vi "CalcPress.vi"(8 "error in (no error)":errorcluster, 10 "Adc_press":i32, 11 "BME68x in":refnum<class "BME680.lvclass">) -> (0 "error out":errorcluster, 2 "Press":i32, 3 "BME68x out":refnum<class "BME680.lvclass">)   [LabVIEW 2022 SP3, in "BME680.lvlib" / "BME680.lvclass"]
uses:
  BME680.lvclass
  BME680.lvclass/BME680.ctl
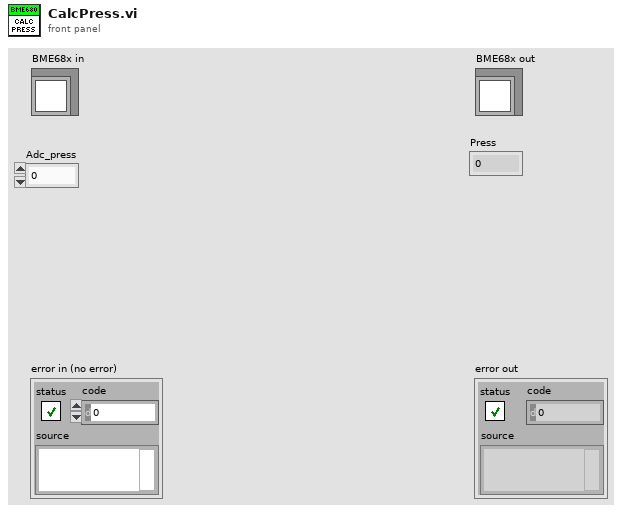
[diagram p1: front panel]
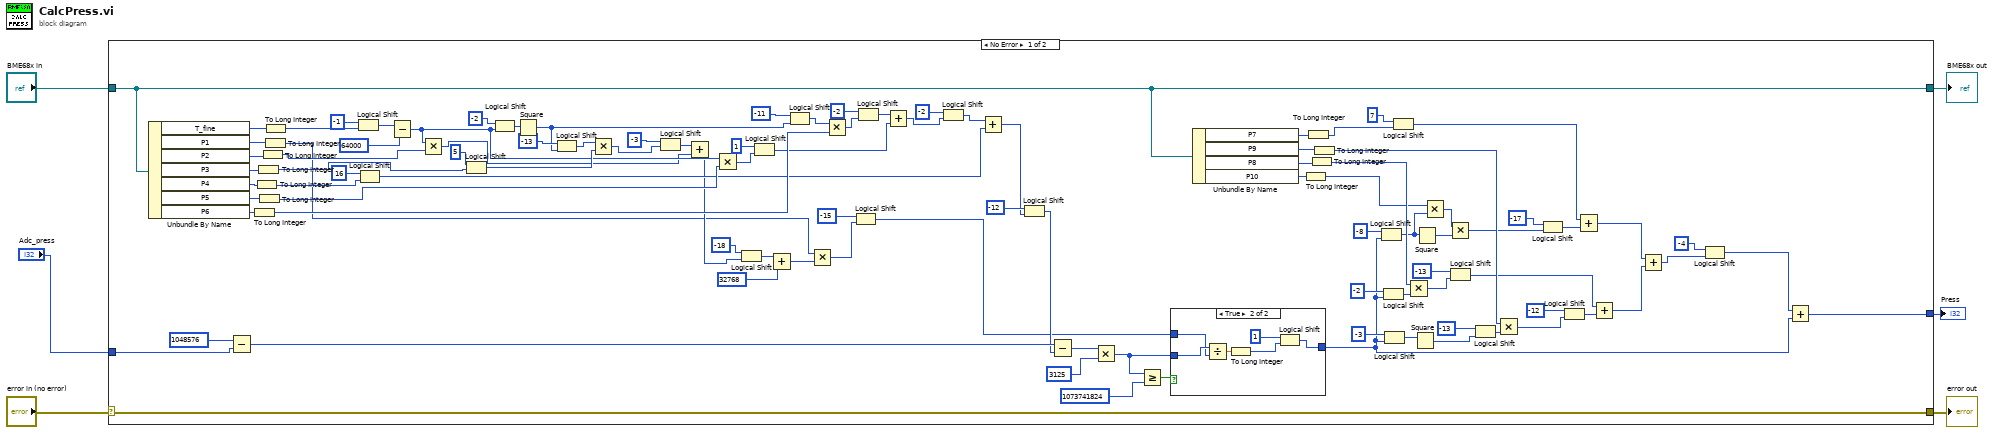
[diagram p0: block diagram]
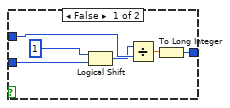
[diagram p2: hidden frame]
diagram:
  n1 = case shown="No Error" "error in (no error)" {
    selector: "error in (no error)" -> [w106 w120]
    tunnel: [w106 w120] -> w5
    tunnel: [w8 w119] -> w3
    tunnel: "BME68x in" -> [w8 w119]
    tunnel: "Adc_press" -> [w55 _]
    tunnel: [w7 _] -> w1
    frame No Error {
      n2 = Unbundle By Name(w8) -> ("T_fine"=w104:i32, "P1"=w105:u16, "P2"=w77:u16, "P3"=w78:u8, "P4"=w82:u16, "P5"=w92:u16, "P6"=w96:u8)
      n3 = Subtract(x=1048576 ("y"), y=w55) -> (x-y=w54:i32)
      n4 = To Long Integer(number=w96) -> (32bit integer=w93:i32)
      n5 = To Long Integer(number=w82) -> (32bit integer=w80:i32)
      n6 = To Long Integer(number=w78) -> (32bit integer=w73:i32)
      n7 = To Long Integer(number=w92) -> (32bit integer=w88:i32)
      n8 = To Long Integer(number=w77) -> (32bit integer=w68:i32)
      n9 = To Long Integer(number=w105) -> (32bit integer=w60:i32)
      n10 = To Long Integer(number=w104) -> (32bit integer=w103:i32)
      n11 = Logical Shift(y=i16 -1, x=w103) -> (x << y=w101:i32)
      n12 = Logical Shift(y=i16 16, x=w80) -> (x << y=w79:i32)
      n13 = Subtract(x=w101, y=64000) -> (x-y=w67:i32)
      n14 = Multiply(x=w67, y=w68) -> (x*y=w65:i32)
      n15 = Logical Shift(y=i16 5, x=w73) -> (x << y=w72:i32)
      n16 = Logical Shift(y=i16 -2, x=w67) -> (x << y=w98:i32)
      n17 = Square(x=w98) -> (x^2=w75:i32)
      n18 = Logical Shift(y=i16 -13, x=w75) -> (x << y=w71:i32)
      n19 = Multiply(x=w71, y=w72) -> (x*y=w69:i32)
      n20 = Logical Shift(y=i16 -3, x=w69) -> (x << y=w66:i32)
      n21 = Add(x=w66, y=w65) -> (x+y=w63:i32)
      n22 = Multiply(x=w67, y=w88) -> (x*y=w87:i32)
      n23 = Logical Shift(y=i16 -18, x=w63) -> (x << y=w62:i32)
      n24 = Logical Shift(y=i16 1, x=w87) -> (x << y=w86:i32)
      n25 = Add(x=w62, y=32768) -> (x+y=w59:i32)
      n26 = Logical Shift(y=i16 -11, x=w75) -> (x << y=w94:i32)
      n27 = Multiply(x=w60, y=w59) -> (x*y=w57:i32)
      n28 = Multiply(x=w94, y=w93) -> (x*y=w91:i32)
      n29 = Logical Shift(y=i16 -15, x=w57) -> (x << y=w45:i32)
      n30 = Logical Shift(y=i16 -2, x=w91) -> (x << y=w90:i32)
      n31 = Add(x=w90, y=w86) -> (x+y=w84:i32)
      n32 = Logical Shift(y=i16 -2, x=w84) -> (x << y=w83:i32)
      n33 = Add(x=w83, y=w79) -> (x+y=w52:i32)
      n34 = Logical Shift(y=i16 -12, x=w52) -> (x << y=w51:i32)
      n35 = Subtract(x=w54, y=w51) -> (x-y=w50:i32)
      n36 = Multiply(x=w50, y=3125) -> (x*y=w46:i32)
      n37 = Greater Or Equal?(x=w46, y=1073741824) -> (x >= y?=w47:bool)
      n38 = case shown="True" w47 {
        tunnel: w46 -> [w111 w115]
        tunnel: w45 -> [w110 w114]
        tunnel: [w107 w113] -> w10
        frame False {
          n39 = Logical Shift(y=i16 1, x=w111) -> (x << y=w109:i32)
          n40 = Divide(x=w109, y=w110) -> (x/y=w108:dbl)
          n41 = To Long Integer(number=w108) -> (32bit integer=w107:i32)
        }
        frame True {
          n42 = Divide(x=w115, y=w114) -> (x/y=w118:dbl)
          n43 = To Long Integer(number=w118) -> (32bit integer=w116:i32)
          n44 = Logical Shift(y=i16 1, x=w116) -> (x << y=w113:i32)
        }
      }
      n45 = Unbundle By Name(w8) -> ("P7"=w21:u8, "P9"=w44:u16, "P8"=w42:u16, "P10"=w43:u8)
      n46 = To Long Integer(number=w43) -> (32bit integer=w25:i32)
      n47 = To Long Integer(number=w21) -> (32bit integer=w16:i32)
      n48 = To Long Integer(number=w42) -> (32bit integer=w31:i32)
      n49 = To Long Integer(number=w44) -> (32bit integer=w33:i32)
      n50 = Logical Shift(y=i16 -8, x=w10) -> (x << y=w24:i32)
      n51 = Logical Shift(y=i16 -2, x=w10) -> (x << y=w32:i32)
      n52 = Logical Shift(y=i16 -3, x=w10) -> (x << y=w40:i32)
      n53 = Logical Shift(y=i16 7, x=w16) -> (x << y=w15:i32)
      n54 = Multiply(x=w31, y=w32) -> (x*y=w29:i32)
      n55 = Square(x=w40) -> (x^2=w37:i32)
      n56 = Square(x=w24) -> (x^2=w27:i32)
      n57 = Multiply(x=w25, y=w24) -> (x*y=w26:i32)
      n58 = Multiply(x=w26, y=w27) -> (x*y=w22:i32)
      n59 = Logical Shift(y=i16 -13, x=w29) -> (x << y=w19:i32)
      n60 = Logical Shift(y=i16 -13, x=w37) -> (x << y=w36:i32)
      n61 = Multiply(x=w33, y=w36) -> (x*y=w35:i32)
      n62 = Logical Shift(y=i16 -17, x=w22) -> (x << y=w18:i32)
      n63 = Logical Shift(y=i16 -12, x=w35) -> (x << y=w20:i32)
      n64 = Add(x=w15, y=w18) -> (x+y=w12:i32)
      n65 = Add(x=w19, y=w20) -> (x+y=w13:i32)
      n66 = Add(x=w12, y=w13) -> (x+y=w11:i32)
      n67 = Logical Shift(y=i16 -4, x=w11) -> (x << y=w9:i32)
      n68 = Add(x=w9, y=w10) -> (x+y=w7:i32)
    }
    frame Error {
    }
  }
  "error out" <- w5
  "BME68x out" <- w3
  "Press" <- w1
